vi "Reached Destination.vi"(8 "error in (no error)":errorcluster, 11 "VISA resource name":refnum<visa-resource-name>) -> (0 "error out":errorcluster, 2 "Done":bool, 3 "VISA resource name out":refnum<visa-resource-name>, 4 "read buffer":string)   [LabVIEW 2019, in "SpectraPro.lvlib"]
uses:
  SpectraPro.lvlib
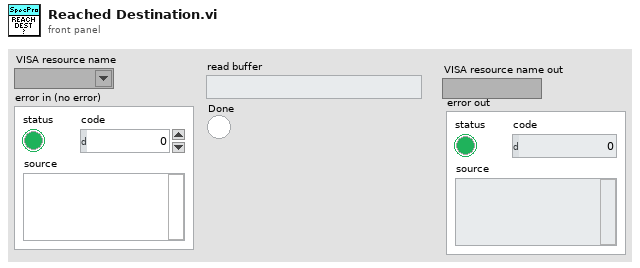
[diagram p1: front panel]
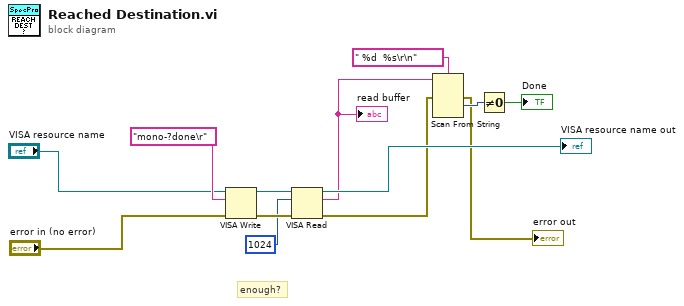
[diagram p0: block diagram]
diagram:
  # "enough?"
  n1 = VISA Write(VISA resource name="VISA resource name", write buffer="mono-?done\r", error in (no error)="error in (no error)") -> (VISA resource name out=w11:refnum<visa-resource-name>, error out=w12:errorcluster)  [unwired: 1 out]
  n2 = VISA Read(VISA resource name=w11, byte count=u32 1024, error in (no error)=w12) -> (VISA resource name out=→"VISA resource name out":refnum<visa-resource-name>, read buffer=w8:string, error out=w2:errorcluster)  [unwired: 1 out]
  "read buffer" <- w8
  n3 = Scan From String(format string=" %d  %s\r\n", input string=w8, error in=w2) -> (error out=→"error out":errorcluster, output 1=w6:i32)  [unwired: 4 in, 2 out]
  n4 = Not Equal To 0?(x=w6) -> (x != 0?=→"Done":bool)
